vi "VI Konfig FT-IR.vi"() -> ()   [LabVIEW 2020, in "FT-IR.lvlib"]
uses:
  Seiten/FT-IR/FT-IR.lvlib
  Visualisierungs Elemente/Zahlen-Ausgabefeld.ctl
  Visualisierungs Elemente/Zahlen-Eingabefeld.ctl
  Visualisierungs Elemente/String - Ausgabefeld.ctl
  Visualisierungs Elemente/Button.ctl
  Visualisierungs Elemente/Auswahlfeld.ctl
  Seiten/FT-IR/1Hz-5Hz Geraet.ctl
  Seiten/FT-IR/xyGraph.ctl
  Seiten/FT-IR/ReadLabFile/Aswahl Lab File.ctl
  Seiten/FT-IR/FGV FT-IR Diagnose Aktionen.ctl
  Seiten/FT-IR/FGV FT-IR Aktionen.ctl
  Seiten/FT-IR/FGV FT-IR Gasliste Aktionen.ctl
  Passwortverwaltung/FGV Passwort Aktion.ctl
  Seiten/FT-IR/ReadLabFile/Aktionen Lab File.ctl
  Seiten/FT-IR/Aktionen EVID-Codes.ctl
  Seiten/FT-IR/Get Spectra/Aktion FGV Background-Daten.ctl
  Messdaten/Aktionen FGV Messdaten.ctl
  Auto Kalibrieren/Aktionen Zeitstempel speichern.ctl
  Seiten/FT-IR/Span/Aktion FGV Span.ctl
  Seiten/FT-IR/Get Spectra/get Spectra.vi
  Allgemein/Diagnose Zykluszeit.vi
  Seiten/FT-IR/Span/VI Span Seite.vi
  Seiten/FT-IR/Konfig Recipes.vi
  Seiten/FT-IR/Algebraic Modul/VI Algebraic Konfig.vi
  Passwortverwaltung/Passwort.lvlib
  Seiten/FT-IR/TOOLweb Interface Library/TOOLweb Interface.lvlib
  Allgemein/allgemeine Sub-VIs.lvlib
  Seiten/Grafik/Grafik.lvlib
  Messdaten/Messdaten.lvlib
  Seiten/Log Konfig/LogKonfig.lvlib
  Seiten/FT-IR/ReadLabFile/Read Lab File.lvlib
  Seiten/FT-IR/Algebraic Modul/Algebraic Modul.lvlib
  cRIO/PC/Kommunikation mit cRIO.lvlib
  Seiten/FT-IR/Get Spectra/Get Spectra.lvlib
  Seiten/FT-IR/Span/Spanfaktor.lvlib
  Auto Kalibrieren/Auto Kalibrieren.lvlib
panel:
  in  "Algebraic":T1
  in  "Average IAG Software:":bool caption="IAG Software:"
  in  "Average":u32=1 caption="Rolling - Average:" min=1 max=600
  in  "Average via AK:":bool caption="AK:"
  in  "Smoothing Aktiv?:":bool
  in  "Komm. Leitsystem:":T2=1 caption="Komm. Leitsystem" items=["1Hz"=1, "5Hz"=5, "10Hz"=10]
  in  "Span":bool caption="FTIR-Diag"
  in  "Rezepte wechseln":bool caption="FTIR-Diag"
  in  "Diagnose Zykluszeit":bool caption="FTIR-Diag"
  in  "FTIR-Diag":bool
  out "Mwert":sgl format="%.3f"
  out "PMwert":sgl format="%.3f"
  in  "Gas 1":T3 items=["NO (350,3000) LP 191C", "NO2 (150) LP 191C (1of2)", "NO2 (2000) LP 191C (2of2)", "N2O (300) LP 191C (1of2)", "NH3 (300) LP 191C (1of2)", "NH3 (900,3000) LP 191C (2of2)", "HNCO (400) 191C", "H2O% (30) LP 191C", "Formaldehyde (70,500) LP 191C", "CO2 low% (4) LP 191C (2of2)", "CO2% (20) LP 191C (1of2)", "CO (700) LP 191C (1of3)", "CO% (1) LP 191C (2of3)", "Propylene (1000) LP 191C", "Aromatic HC C7 (500) LP 191C", "Ethylene (1000) LP 191C", "CH4 (250) LP 191C (1of2)", "CH4 (5000) LP 191C (2of2)", "Ethane (1000) LP 191C", "Acetylene (1000) LP 191C", "HNO2 (20) 191C", "MeOH (1000) 191C", "CO% (10) LP 191C (3of3)", "Formic Acid (100) 191C", "SO2 (500) LP 191C", "Acetaldehyde (1000) LP 191C", "COS (100) LP 191C", "1,3 butadiene (100) LP 191C", "Oil as Octane (200) LP 191C", "N2O (1000) LP 191C (2of2)", "Propane (200) LP 191C", "NO2 autorange (2000)", "CO autorange (100000)", "CH4 autorange (5000)", "NH3 autorange (3000)", "NOx autorange (3000)", "HCD (10000)", "NMHCD (10000)", "CO2% autorange (20)", "H2Oppm (300000)", "N2O autorange (1000)", "NMNEHCD (3000)", "Temp. Messzelle", "Druck Messzelle", "sBeam@2500", "Temp. HL zu FT-IR", "Temp. HL Extern SP1", "Austrittstemp. FT-IR", "Temp. Schaltschrank", "Konstant 0", "Konstant 50", "Konstant 100", "AK DUMMY"]
  out "Konzentration 1":T4 format="%.3f"
  out "Graph 1":waveform(dbl)(graph)
  in  "Auswahl":T5
  out "Zeitstempel":timestamp
  out "Graph":T6 caption="Graph 2"
  out "Zykluszeit":T4 caption="Zykluszeit:" format="%.3f"
  in  "Gerätetype:":T2=1 items=["1Hz"=1, "5Hz"=5, "10Hz"=10]
  out "Zeitstempeln":timestamp[](array[timestamp]) format="%<%H:%M:%S\n%x>T"
  in  "Anzahl":i32=1
  in  "Startadresse":i32=11000
  out "Betriebsstunden FT-IR":T4 format="%.1f"
  out "Aktuelles Rezept":T7
  in  "Gasliste vergleichen":T1
  out "Aktuelle Gasliste":T7[](array[typedef])
  out "(1) InstrumentState":T7
  in  "(90) ftirScans":T8 format="%#_5g"
  out "(10) NrOfGasses":T4 format="%#_5g"
  in  "FT-IR MAX":T9 {"Max sBeam" format="%#_5g"; "Max LinCheck" format="%#_5g"; "Max LaserPP" format="%#_5g"}
  in  "FT-IR MIN":T10 {"Min sBeam" format="%#_5g"; "Min LinCheck" format="%#_5g"; "Min LaserPP" format="%#_5g"}
  out "Ist sBeam":T4 format="%.2f"
  out "Ist LinCheck":T4 format="%.4f"
  out "Ist LaserPP":T4 format="%.2f"
  # "Konfiguration FT-IR"
  # "Diagnose FT-IR"
  # "Istwert"
  # "Minimaler Wert"
  # "Maximaler Wert"
  # "Aktuelle Gasliste"
  # "Laser PP:"
  # "Linearizer Check:"
  # "sBeam@2500"
  # "Allgemeine Parameter"
  # "Messwerte"
  # "Hintergrund Spectrum"
  # "sec"
  # "±"
  # "x"
  # "Zykluszeit:"
  # "sec"
  # "Letzte Kalibrierung:"
  # "Algebraic (EVID Code):"
  # "Startadresse:"
  # "Anzahl:"
  # "Betriebsstunden FT-IR:"
  # "Aktuelles Rezept:"
  # "Instrument State:"
  # "Number of Scan:"
  # "Number of Gases:"
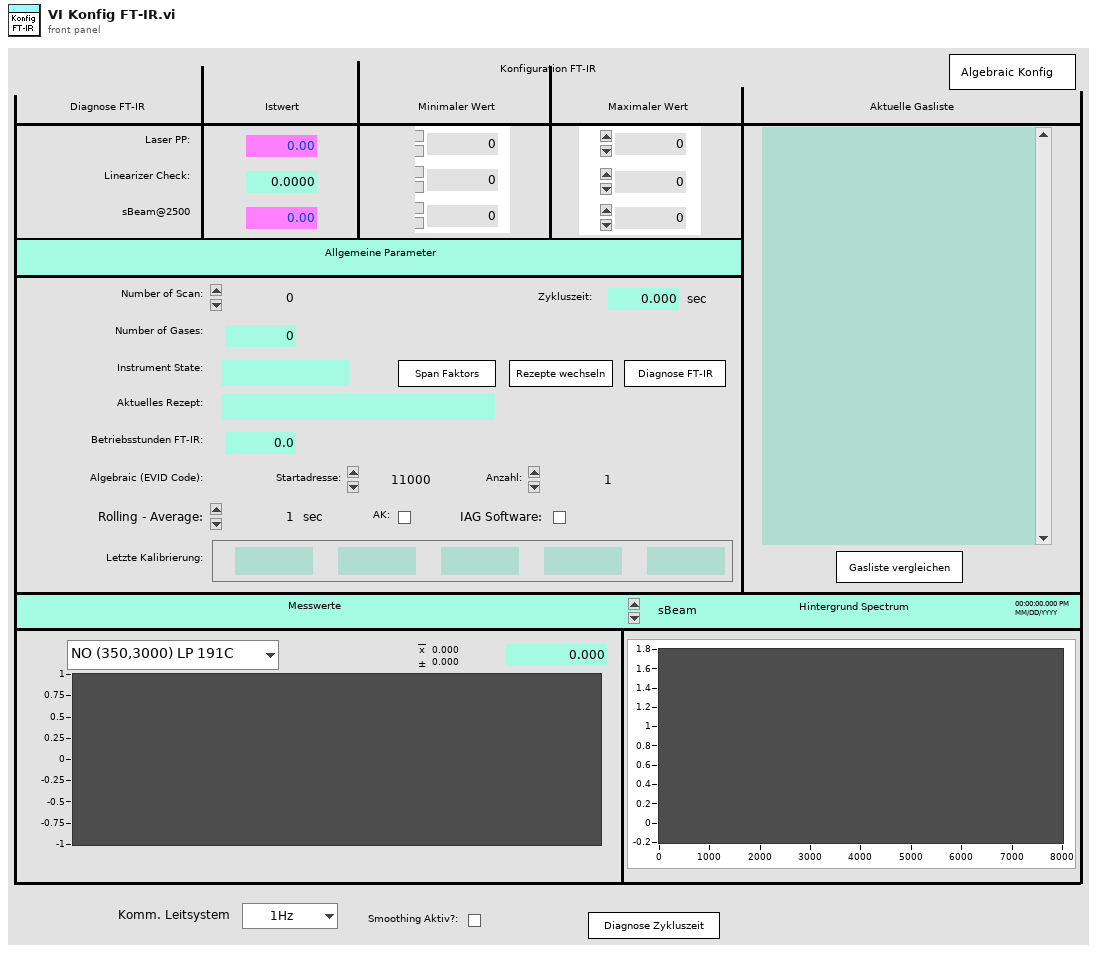
[diagram p1: front panel]
types:
  T1 = typedef "Button.ctl" = bool
  T2 = typedef "FT-IR.lvlib/1Hz-5Hz Geraet.ctl" = u16
  T3 = typedef "Auswahlfeld.ctl" = u16
  T4 = typedef "Zahlen-Ausgabefeld.ctl" = sgl
  T5 = typedef "FT-IR.lvlib/Read Lab File.lvlib/Aswahl Lab File.ctl" = enum16{"sBeam", "Main", "igram", "Previous"}
  T6 = typedef "FT-IR.lvlib/xyGraph.ctl" = cluster{dbl[], "Y":dbl[]}[]
  T7 = typedef "String - Ausgabefeld.ctl" = string
  T8 = typedef "Zahlen-Eingabefeld.ctl" = sgl
  T9 = cluster{"Max LaserPP":T8, "Max LinCheck":T8, "Max sBeam":T8}
  T10 = cluster{"Min LaserPP":T8, "Min LinCheck":T8, "Min sBeam":T8}
  T11 = typedef "FT-IR.lvlib/Get Spectra.lvlib/Aktion FGV Background-Daten.ctl" = enum16{"lesen", "schreiben", "Background aktiv", "Referenz", "laden", "speichern", "Plot sichtbar"}
  T12 = enum8{"Enabled", "Disabled", "Disabled and Grayed Out"}
  T13 = typedef "FT-IR.lvlib/Aktionen EVID-Codes.ctl" = enum16{"lesen", "setzen", "laden", "speichern", "1Hz/5Hz", "Smoothing", "Rolling Average"}
  T14 = typedef "FT-IR.lvlib/Read Lab File.lvlib/Aktionen Lab File.ctl" = enum16{"lesen", "laden"}
  T15 = typedef "Passwort.lvlib/FGV Passwort Aktion.ctl" = enum16{"prüfen", "setzen", "Initialisieren", "PW speichern", "lesen", "PW Änderung"}
  T16 = typedef "FT-IR.lvlib/FGV FT-IR Gasliste Aktionen.ctl" = enum16{"lesen", "Gasliste FT-IR", "Gasliste ausgelesen", "laden", "speichern", "löschen"}
  T17 = typedef "FT-IR.lvlib/FGV FT-IR Aktionen.ctl" = enum16{"lesen", "NOG setzen", "NOS setzen", "Initialisieren", "speichern", "ALLES setzen", "FT-IR Spektrum loggen", "Komm Stoppen", "Spektrum LogKonfig"}
  T18 = typedef "FT-IR.lvlib/FGV FT-IR Diagnose Aktionen.ctl" = enum16{"Lesen", "Diagnose Schreiben", "Min Schreiben", "Max Schreiben"}
  T19 = typedef "FT-IR.lvlib/Rolling Average Settings.ctl" = cluster{"Average":u32, "Average via AK:":bool, "Average IAG Software:":bool}
  T20 = cluster{"LaserPP Max":dbl, "LinCheck Max":dbl, "sBeam Max":dbl}
  T21 = cluster{"LaserPP Min":dbl, "LinCheck Min":dbl, "sBeam Min":dbl}
  T22 = typedef "Auto Kalibrieren.lvlib/Aktionen Zeitstempel speichern.ctl" = enum16{"lesen", "Zeitstempel NEU", "laden", "speichern"}
  T23 = typedef "Messdaten.lvlib/Aktionen FGV Messdaten.ctl" = enum16{"lesen", "schreiben", "löschen", "Mittelwerte", "Komponente"}
  T24 = typedef "FT-IR.lvlib/Spanfaktor.lvlib/Aktion FGV Span.ctl" = enum16{"lesen", "Span", "Seite aktiv", "Offset", "FGV aktualisiert", "Aktualisierung aufheben"}
  T25 = typedef "FT-IR.lvlib/TOOLweb Interface.lvlib/Typdefinitionen.lvlib/TOOLweb Diagnose.ctl" = cluster{"(14) temperature":sgl, "(15) pressure":sgl, "(16) oxygen":sgl, "(50) diag-igramdc":sgl, "(51) diag-igrampp":sgl, "(52) diag-phaseAngle":sgl, "(53) diag-laserpp":sgl, "(54) diag-laserdc":sgl, "(55) diag-badscan":sgl, "(56) diag-centerburst":sgl, "(57) diag-linearizerCheck":sgl, "(58) diag-SNR":sgl, "(59) diag-sBeamIntensity":sgl}
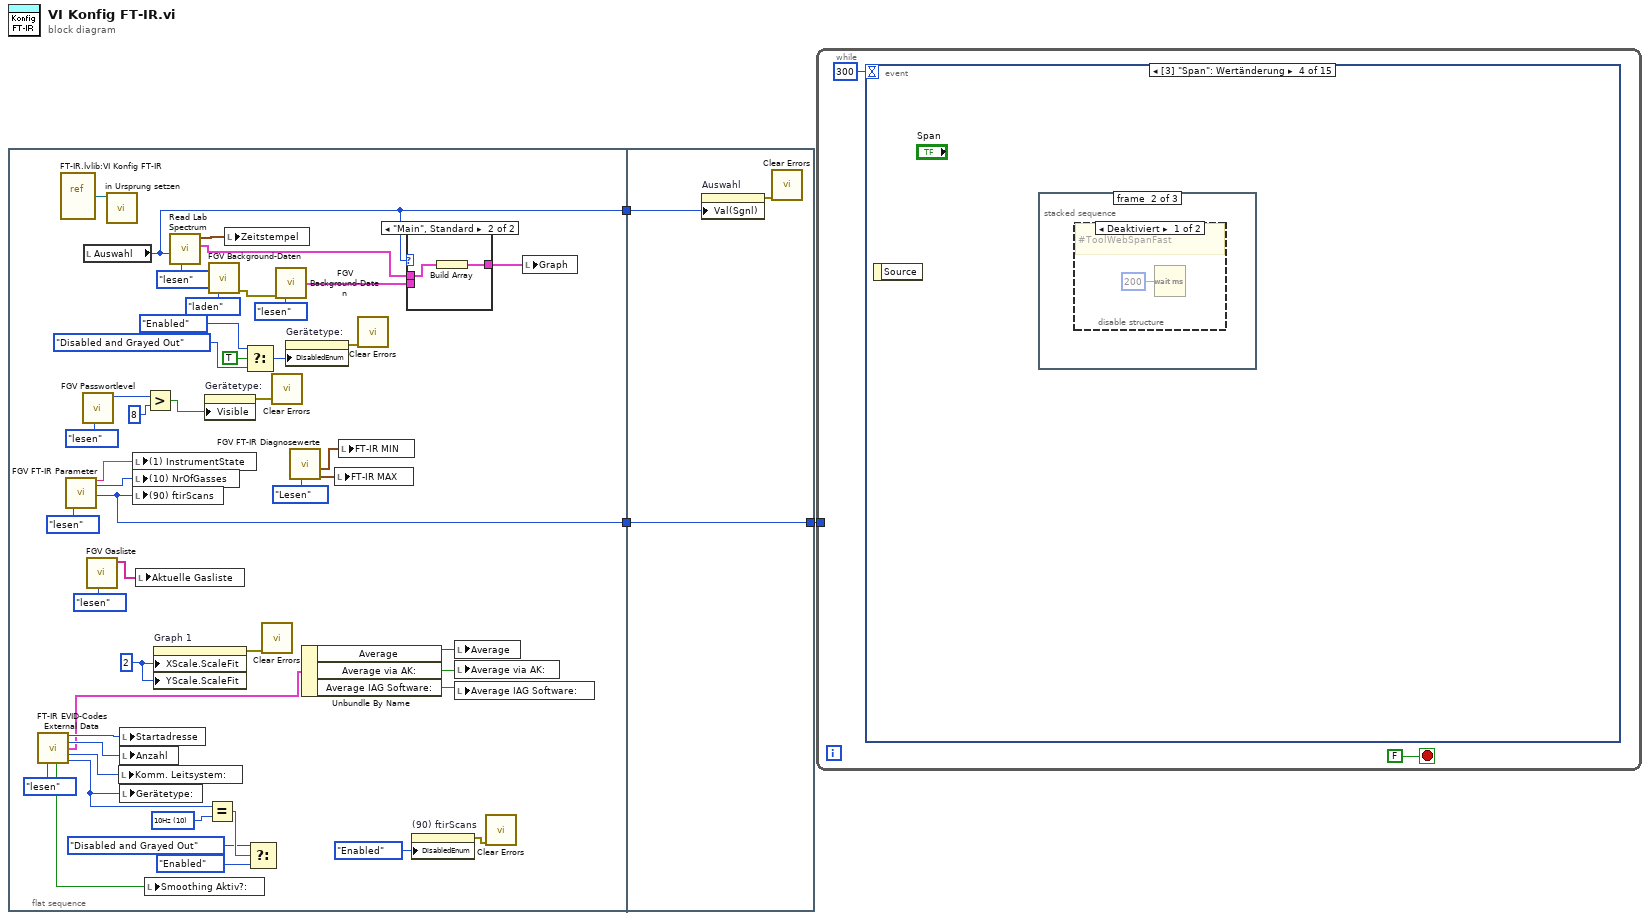
[diagram p0: block diagram]
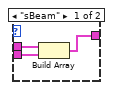
[diagram p2: hidden frame]
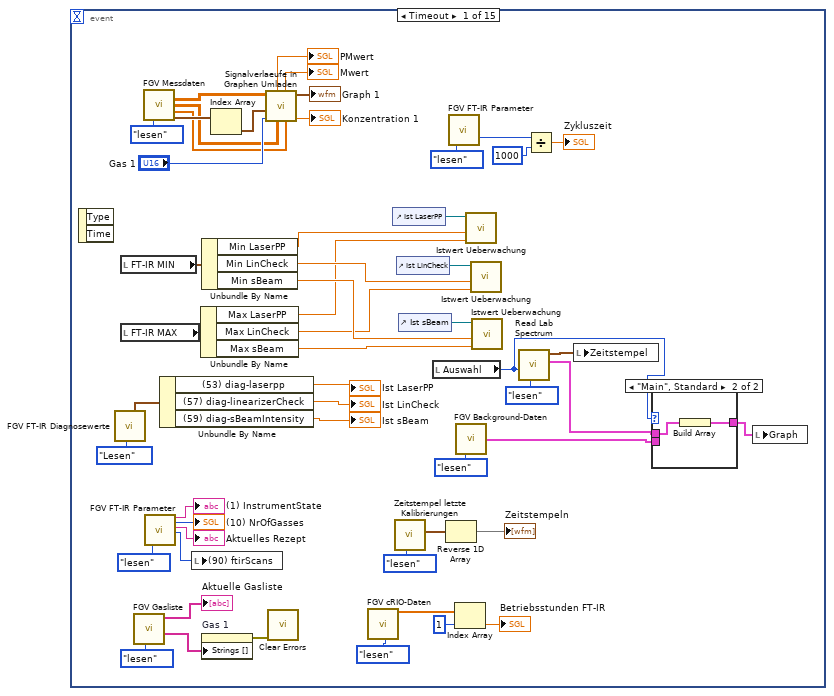
[diagram p3: hidden frame]
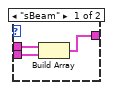
[diagram p4: hidden frame]
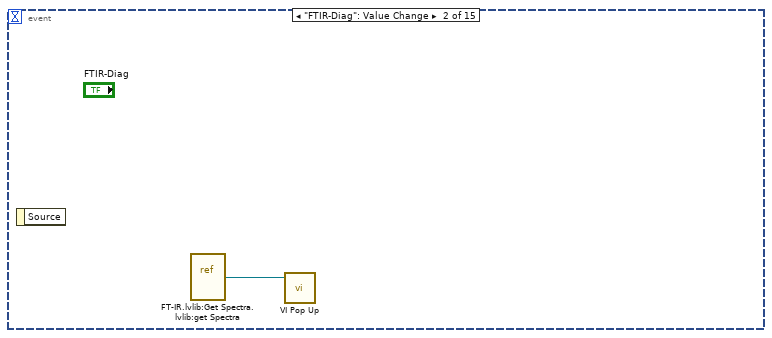
[diagram p5: hidden frame]
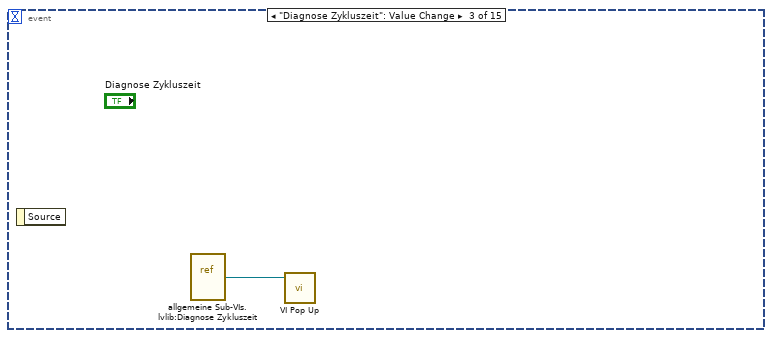
[diagram p6: hidden frame]
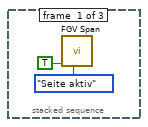
[diagram p7: hidden frame]
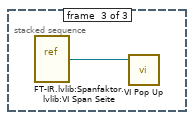
[diagram p9: hidden frame]
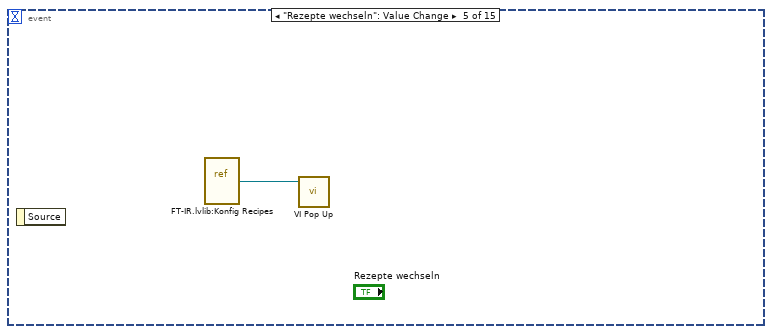
[diagram p10: hidden frame]
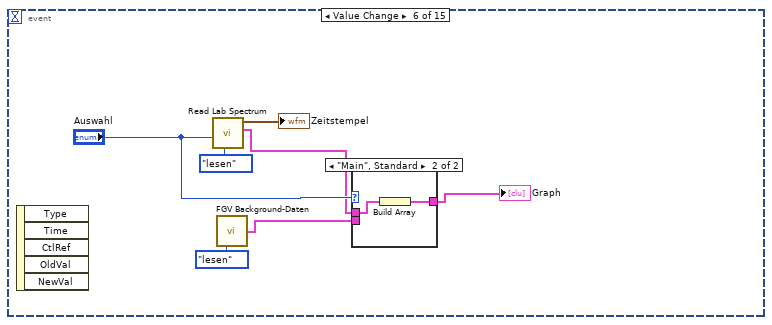
[diagram p11: hidden frame]
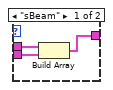
[diagram p12: hidden frame]
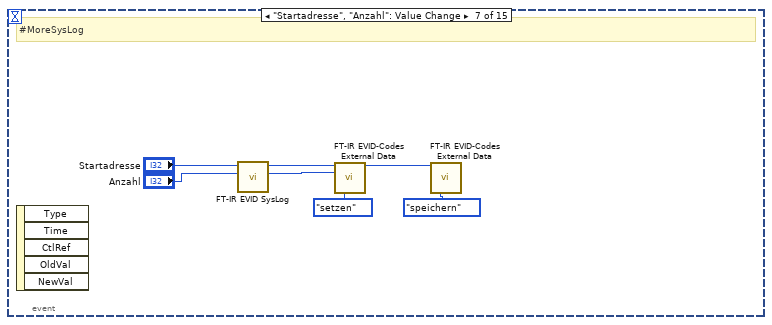
[diagram p13: hidden frame]
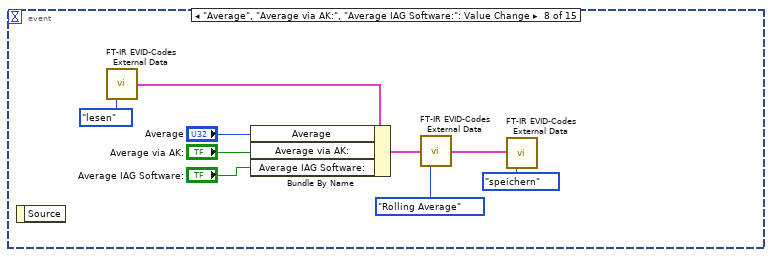
[diagram p14: hidden frame]
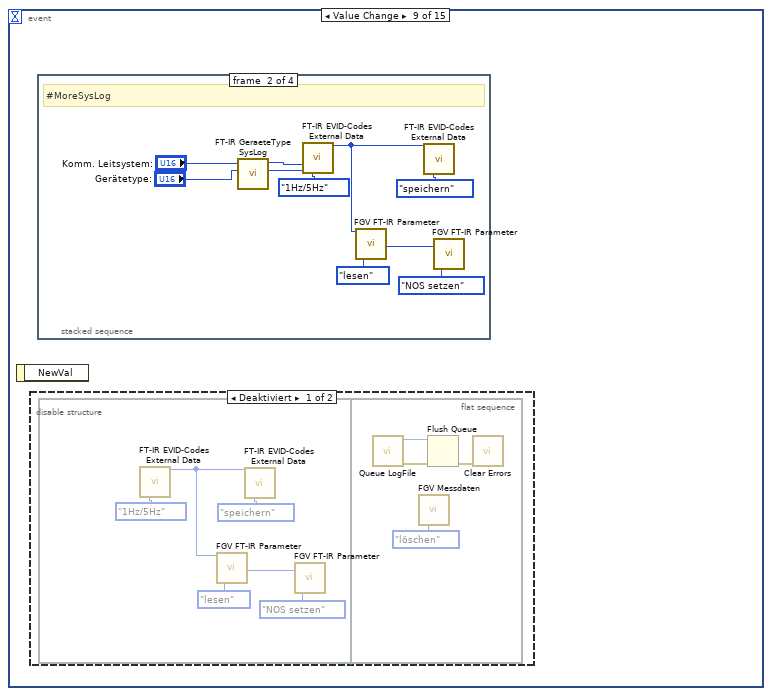
[diagram p15: hidden frame]
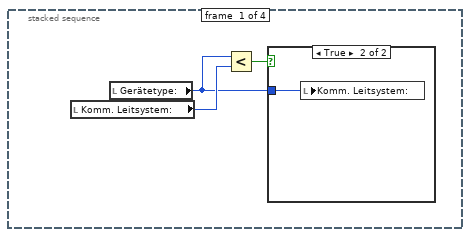
[diagram p17: hidden frame]
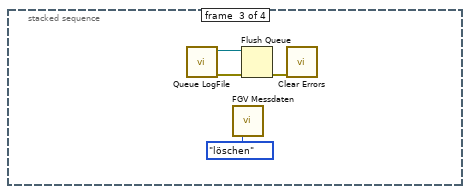
[diagram p19: hidden frame]
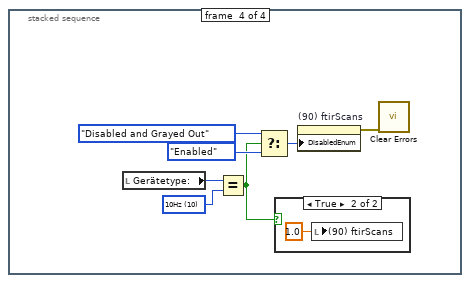
[diagram p20: hidden frame]
diagram:
  n1 = flat-sequence {
    tunnel: [w44] -> w3
    tunnel: [w5] -> w2
    tunnel: [w58] -> w1
    tunnel: w3 -> [w58]
    tunnel: w2 -> [w57]
    frame #0 {
      w23 = T2 10 items=["1Hz"=1, "5Hz"=5, "10Hz"=10] ("y")
      w42 = u8 2 ("X-Achse.Achsenanpassung")
      n2 = call "FT-IR EVID-Codes External Data.vi"("Aktionen"=Aktionen_EVID-Codes."lesen") -> ("Startadresse"=w26:i32, "Anzahl"=w27:i32, "Rolling Average Settings"=w16:T19, "1Hz/5Hz Leitsystem"=w19:T2, "Smoothing?"=w17:bool, "1Hz/5Hz Gerät"=w20:T2)  [unwired: 9 in]
      n3 = vi-ref "FT-IR.lvlib:VI Konfig FT-IR.vi"() -> (w32:refnum<vi>)
      n4 = call "FGV FT-IR Parameter.vi"("Aktion"=FGV_FT-IR_Aktionen."lesen") -> ("Instrument State"=w45:string, "NoOfGasses"=w46:u32, "NoOfScan"=w44:u32)  [unwired: 11 in, 5 out]
      n5 = call "FGV Passwortlevel.vi"("FGV Passwort Aktion"=FGV_Passwort_Aktion."lesen") -> ("aktueller Level"=w40:i16)  [unwired: 3 in, 7 out]
      n6 = local read "Auswahl"() -> (w5:T5)
      n7 = call "FGV Gasliste.vi"("Aktionen"=FGV_FT-IR_Gasliste_Aktionen."lesen") -> ("Aktuelle Gasliste FT-IR"=w30:T7[])  [unwired: 8 in, 2 out]
      n8 = call "in Ursprung setzen.vi"("VI Referenz"=w32) -> ()  [unwired: 10 in, 1 out]
      n9 = local write "Komm. Leitsystem:"(w19) -> ()
      n10 = local write "Startadresse"(w26) -> ()
      n11 = local write "Anzahl"(w27) -> ()
      n12 = local write "Gerätetype:"(w20) -> ()
      n13 = local write "(1) InstrumentState"(w45) -> ()
      n14 = local write "(10) NrOfGasses"(w46) -> ()
      n15 = local write "(90) ftirScans"(w44) -> ()
      n16 = local write "Aktuelle Gasliste"(w30) -> ()
      n17 = Greater?(x=w40, y=i16 8) -> (0:w29:bool)
      n18 = local write "Smoothing Aktiv?:"(w17) -> ()
      n19 = property on="Graph 1" class="SVDiagr (strikt)"("XScale.ScaleFit"=w42, "YScale.ScaleFit"=w42) -> (error out=w36:errorcluster)  [unwired: 2 in, 1 out]
      n20 = call "Read Lab Spectrum.VI"("Aktionen"=Aktionen_Lab_File."lesen", "Auswahl"=w5) -> ("Graph"=w9:cluster{dbl[], sgl[]}, "Zeitstempel"=w12:timestamp)  [unwired: 6 in, 2 out]
      n21 = property on="Gerätetype:" class="Ring (strikt)"("Visible"=w29) -> (error out=w28:errorcluster)  [unwired: 2 in, 1 out]
      n22 = Equal?(x=w20, y=w23) -> (x = y?=w24:bool)
      n23 = call "FGV Background-Daten.vi"("Aktion"=Aktion_FGV_Background-Daten."laden") -> ("error out"=w6:errorcluster)  [unwired: 7 in, 7 out]
      n24 = local write "Zeitstempel"(w12) -> ()
      n25 = Select(t=T12."Enabled", s=TRUE, f=T12."Disabled and Grayed Out" ("Deaktiviert")) -> (s? t:f=w33:T12)
      n26 = Select(t=T12."Disabled and Grayed Out" ("Deaktiviert"), s=w24, f=T12."Enabled" ("t")) -> ()  [unwired: 1 out]
      n27 = call <vilib>:"Clear Errors.vi"("error in (no error)"=w36) -> ()  [unwired: 5 in, 2 out]
      n28 = call <vilib>:"Clear Errors.vi"("error in (no error)"=w28) -> ()  [unwired: 5 in, 2 out]
      n29 = call "FGV Background-Daten.vi"("error in (no error)"=w6, "Aktion"=Aktion_FGV_Background-Daten."lesen") -> ("Referenz-200"=w4:cluster{"Ramp Pattern":dbl[], dbl[]})  [unwired: 6 in, 7 out]
      n30 = property on="Gerätetype:" class="Ring (strikt)"("DisabledEnum"=w33) -> (error out=w37:errorcluster)  [unwired: 2 in, 1 out]
      n31 = call "FGV FT-IR Diagnosewerte.vi"("Aktionen"=FGV_FT-IR_Diagnose_Aktionen."Lesen") -> ("FT-IR MAX"=w50:T20, "FT-IR MIN"=w49:T21)  [unwired: 5 in, 4 out]
      n32 = Unbundle By Name(w16) -> ("Average"=w15:u32, "Average via AK:"=w14:bool, "Average IAG Software:"=w13:bool)
      n33 = local write "FT-IR MAX"(w50) -> ()
      n34 = local write "FT-IR MIN"(w49) -> ()
      n35 = call <vilib>:"Clear Errors.vi"("error in (no error)"=w37) -> ()  [unwired: 5 in, 2 out]
      n36 = case shown="\"Main\", Standard" w5 {
        tunnel: w4 -> [w53 _]
        tunnel: w9 -> [w52 w55]
        tunnel: [w51 w54] -> w8
        frame "sBeam" {
          n37 = Build Array(w52, w53) -> (w51:cluster{"Ramp Pattern":dbl[], dbl[]}[])
        }
        frame "Main", Default {
          n38 = Build Array(w55) -> (w54:cluster{dbl[], sgl[]}[])
        }
      }
      n39 = property on="(90) ftirScans" class="DigWert (strikt)"("DisabledEnum"=T12."Enabled" ("Deaktiviert")) -> (error out=w18:errorcluster)  [unwired: 2 in, 1 out]
      n40 = local write "Average"(w15) -> ()
      n41 = local write "Average via AK:"(w14) -> ()
      n42 = local write "Average IAG Software:"(w13) -> ()
      n43 = call <vilib>:"Clear Errors.vi"("error in (no error)"=w18) -> ()  [unwired: 5 in, 2 out]
      n44 = local write "Graph"(w8) -> ()
    }
    frame #1 {
      n45 = property on="Auswahl" class="Enum (strikt)"("Val(Sgnl)"=w57) -> (error out=w56:errorcluster)  [unwired: 2 in, 1 out]
      n46 = call <vilib>:"Clear Errors.vi"("error in (no error)"=w56) -> ()  [unwired: 5 in, 2 out]
    }
  }
  n47 = while {
    tunnel: w1 -> [_]
    stop <- FALSE stop-if-true
    n48 = event shown="[3] \"Span\": Wertänderung" {
      selector: _ -> [_ _ _ _ _ _ _ _ _ _ _ _ _ _ _]
      dyn-events: _ -> [_ _ _ _ _ _ _ _ _ _ _ _ _ _ _]
      timeout: 300 -> [_ _ _ _ _ _ _ _ _ _ _ _ _ _ _]
      event Timeout {
        n49 = event-data() -> ()  [unwired: 1 in, 2 out]
        n50 = call "FGV FT-IR Diagnosewerte.vi"("Aktionen"=FGV_FT-IR_Diagnose_Aktionen."Lesen") -> ("Diagnose"=w103:T25)  [unwired: 5 in, 5 out]
        n51 = local read "FT-IR MIN"() -> (w107:T10)
        n52 = local read "FT-IR MAX"() -> (w108:T9)
        n53 = call "FGV Gasliste.vi"("Aktionen"=FGV_FT-IR_Gasliste_Aktionen."lesen") -> ("Aktuelle Gasliste gesamt"=w73:T7[], "Aktuelle Gasliste FT-IR"=→"Aktuelle Gasliste":T7[])  [unwired: 8 in, 1 out]
        n54 = call "FGV Messdaten.vi"("Aktionen"=Aktionen_FGV_Messdaten."lesen") -> ("Messdaten"=w74:sgl[][], "Mittelwertdaten"=w72:sgl[][], "Deviation"=w71:sgl[], "Zeitstempeln"=w88:timestamp[])  [unwired: 6 in, 5 out]
        n55 = call "FGV FT-IR Parameter.vi"("Aktion"=FGV_FT-IR_Aktionen."lesen") -> ("Instrument State"=→"(1) InstrumentState":string, "NoOfGasses"=→"(10) NrOfGasses":u32, "Current Recipe"=→"Aktuelles Rezept":string, "NoOfScan"=w68:u32)  [unwired: 11 in, 4 out]
        n56 = Unbundle By Name(w103) -> ("(53) diag-laserpp"=→"Ist LaserPP":sgl, "(57) diag-linearizerCheck"=→"Ist LinCheck":sgl, "(59) diag-sBeamIntensity"=→"Ist sBeam":sgl)
        n57 = local write "(90) ftirScans"(w68) -> ()
        n58 = Unbundle By Name(w108) -> ("Max LaserPP"=w110:T8, "Max LinCheck"=w112:T8, "Max sBeam"=w114:T8)
        n59 = Unbundle By Name(w107) -> ("Min LaserPP"=w109:T8, "Min LinCheck"=w111:T8, "Min sBeam"=w113:T8)
        n60 = property on="Gas 1" class="Ring (strikt)"("Strings []"=w73) -> (error out=w75:errorcluster)  [unwired: 2 in, 1 out]
        n61 = Index Array(array=w88) -> (element=w86:timestamp)  [unwired: 1 in]
        n62 = call "Signalverlaeufe in Graphen Umladen.vi"("Deviation"=w71, "Mittelwertdaten"=w72, "Gas-Auswahl"="Gas 1", "t0"=w86, "Werte"=w74) -> ("Konzentration"=→"Konzentration 1":sgl, "Waveform"=→"Graph 1":waveform(dbl), "aktuelle Mittelwert"=→"Mwert":sgl, "Deviation"=→"PMwert":sgl)  [unwired: 2 in, 1 out]
        n63 = call <vilib>:"Clear Errors.vi"("error in (no error)"=w75) -> ()  [unwired: 5 in, 2 out]
        n64 = call "FGV cRIO-Daten.vi"("Aktion"=enum16{"lesen", "schreiben"}."lesen") -> ("Betriebsstunden"=w76:sgl[])  [unwired: 9 in, 9 out]
        n65 = control-ref of="Ist LaserPP"() -> (w104:refnum<vi>)
        n66 = call "Zeitstempel letzte Kalibrierungen.vi"("Aktionen"=Aktionen_Zeitstempel_speichern."lesen") -> ("Zeitstempeln"=w66:timestamp[])  [unwired: 10 in]
        n67 = control-ref of="Ist LinCheck"() -> (w105:refnum<vi>)
        n68 = control-ref of="Ist sBeam"() -> (w106:refnum<vi>)
        n69 = local read "Auswahl"() -> (w62:T5)
        n70 = Reverse 1D Array(array=w66) -> (reversed array=→"Zeitstempeln":timestamp[])
        n71 = call "FGV FT-IR Parameter.vi"("Aktion"=FGV_FT-IR_Aktionen."lesen") -> ("Zykluszeit Messdatenverteiler"=w82:u32)  [unwired: 11 in, 7 out]
        n72 = Index Array(array=w76, index=1 ("Index")) -> (element=→"Betriebsstunden FT-IR":sgl)
        n73 = call "FGV Background-Daten.vi"("Aktion"=Aktion_FGV_Background-Daten."lesen") -> ("Referenz-200"=w61:cluster{"Ramp Pattern":dbl[], dbl[]})  [unwired: 7 in, 7 out]
        n74 = call "Istwert Ueberwachung.vi"("Max"=w110, "Min"=w109, "Referernz"=w104) -> ()  [unwired: 9 in]
        n75 = call "Istwert Ueberwachung.vi"("Max"=w112, "Min"=w111, "Referernz"=w105) -> ()  [unwired: 9 in]
        n76 = call "Istwert Ueberwachung.vi"("Max"=w114, "Min"=w113, "Referernz"=w106) -> ()  [unwired: 9 in]
        n77 = call "Read Lab Spectrum.VI"("Aktionen"=Aktionen_Lab_File."lesen", "Auswahl"=w62) -> ("Graph"=w64:cluster{dbl[], sgl[]}, "Zeitstempel"=w70:timestamp)  [unwired: 6 in, 2 out]
        n78 = Divide(x=w82, y=u32 1000) -> (x/y=→"Zykluszeit":dbl)
        n79 = local write "Zeitstempel"(w70) -> ()
        n80 = case shown="\"Main\", Standard" w62 {
          tunnel: w61 -> [w117 _]
          tunnel: w64 -> [w116 w119]
          tunnel: [w115 w118] -> w63
          frame "sBeam" {
            n81 = Build Array(w116, w117) -> (w115:cluster{"Ramp Pattern":dbl[], dbl[]}[])
          }
          frame "Main", Default {
            n82 = Build Array(w119) -> (w118:cluster{dbl[], sgl[]}[])
          }
        }
        n83 = local write "Graph"(w63) -> ()
      }
      event "FTIR-Diag": Value Change {
        n84 = event-data() -> ()  [unwired: 1 in, 1 out]
        n85 = vi-ref "FT-IR.lvlib:Get Spectra.lvlib:get Spectra.vi"() -> (w120:refnum<vi>)
        n86 = call "VI Pop Up.vi"("VI Referenz"=w120) -> ()  [unwired: 10 in, 1 out]
      }
      event "Diagnose Zykluszeit": Value Change {
        n87 = event-data() -> ()  [unwired: 1 in, 1 out]
        n88 = vi-ref "allgemeine Sub-VIs.lvlib:Diagnose Zykluszeit.vi"() -> (w121:refnum<vi>)
        n89 = call "VI Pop Up.vi"("VI Referenz"=w121) -> ()  [unwired: 10 in, 1 out]
      }
      event "Span": Value Change {
        n90 = event-data() -> ()  [unwired: 1 in, 1 out]
        n91 = stacked-sequence {
          frame #0 {
            n92 = call "FGV Span.vi"("Aktion"=Aktion_FGV_Span."Seite aktiv", "Aktiv"=TRUE) -> ()  [unwired: 6 in, 4 out]
          }
          frame #1 {
            n93 = disable-structure shown="Deaktiviert" {
              frame Disabled {
                # "#ToolWebSpanFast"
                n94 = Wait (ms)(milliseconds to wait=u32 200 ("Zu wartende ms")) -> ()  [unwired: 1 out]
              }
              frame Enabled {
              }
            }
          }
          frame #2 {
            n95 = vi-ref "FT-IR.lvlib:Spanfaktor.lvlib:VI Span Seite.vi"() -> (w125:refnum<vi>)
            n96 = call "VI Pop Up.vi"("VI Referenz"=w125) -> ()  [unwired: 10 in, 1 out]
          }
        }
      }
      event "Rezepte wechseln": Value Change {
        n97 = event-data() -> ()  [unwired: 1 in, 1 out]
        n98 = vi-ref "FT-IR.lvlib:Konfig Recipes.vi"() -> (w126:refnum<vi>)
        n99 = call "VI Pop Up.vi"("VI Referenz"=w126) -> ()  [unwired: 10 in, 1 out]
      }
      event Value Change {
        n100 = event-data() -> ()  [unwired: 1 in, 5 out]
        n101 = call "Read Lab Spectrum.VI"("Aktionen"=Aktionen_Lab_File."lesen", "Auswahl"="Auswahl") -> ("Graph"=w130:cluster{dbl[], sgl[]}, "Zeitstempel"=→"Zeitstempel":timestamp)  [unwired: 6 in, 2 out]
        n102 = call "FGV Background-Daten.vi"("Aktion"=Aktion_FGV_Background-Daten."lesen") -> ("Referenz-200"=w127:cluster{"Ramp Pattern":dbl[], dbl[]})  [unwired: 7 in, 7 out]
        n103 = case shown="\"Main\", Standard" "Auswahl" {
          tunnel: w127 -> [w136 _]
          tunnel: w130 -> [w135 w138]
          tunnel: [w134 w137] -> w128
          frame "sBeam" {
            n104 = Build Array(w135, w136) -> (w134:cluster{"Ramp Pattern":dbl[], dbl[]}[])
          }
          frame "Main", Default {
            n105 = Build Array(w138) -> (w137:cluster{dbl[], sgl[]}[])
          }
        }
        "Graph" <- w128
      }
      event "Startadresse", "Anzahl": Value Change {
        # "#MoreSysLog"
        n106 = event-data() -> ()  [unwired: 1 in, 5 out]
        n107 = call "FT-IR EVID SysLog.vi"("Anzahl"="Anzahl", "Startadresse"="Startadresse") -> ("Anzahl out"=w139:i32, "Startadresse out"=w141:i32)  [unwired: 8 in]
        n108 = call "FT-IR EVID-Codes External Data.vi"("Startadresse"=w141, "Anzahl"=w139, "Aktionen"=Aktionen_EVID-Codes."setzen") -> ("Startadresse"=w143:i32)  [unwired: 7 in, 5 out]
        n109 = call "FT-IR EVID-Codes External Data.vi"("Startadresse"=w143, "Aktionen"=Aktionen_EVID-Codes."speichern") -> ()  [unwired: 8 in, 6 out]
      }
      event "Average", "Average via AK:", "Average IAG Software:": Value Change {
        n110 = event-data() -> ()  [unwired: 1 in, 1 out]
        n111 = call "FT-IR EVID-Codes External Data.vi"("Aktionen"=Aktionen_EVID-Codes."lesen") -> ("Rolling Average Settings"=w153:T19)  [unwired: 9 in, 5 out]
        n112 = Bundle By Name(cluster=w153, "Average"="Average", "Average via AK:"="Average via AK:", "Average IAG Software:"="Average IAG Software:") -> (w148:T19)
        n113 = call "FT-IR EVID-Codes External Data.vi"("Rolling Average Settings"=w148, "Aktionen"=Aktionen_EVID-Codes."Rolling Average") -> ("Rolling Average Settings"=w146:T19)  [unwired: 8 in, 5 out]
        n114 = call "FT-IR EVID-Codes External Data.vi"("Rolling Average Settings"=w146, "Aktionen"=Aktionen_EVID-Codes."speichern") -> ()  [unwired: 8 in, 6 out]
      }
      event Value Change {
        n115 = event-data() -> ()  [unwired: 1 in, 1 out]
        n116 = disable-structure shown="Deaktiviert" {
          frame Disabled {
            n117 = flat-sequence {
              frame #0 {
                n118 = call "FT-IR EVID-Codes External Data.vi"("Aktionen"=Aktionen_EVID-Codes."1Hz/5Hz") -> ("Startadresse"=w155:i32)  [unwired: 9 in, 5 out]
                n119 = call "FGV FT-IR Parameter.vi"("NoOfGasses neu"=w155, "Aktion"=FGV_FT-IR_Aktionen."lesen") -> ("NoOfScan"=w156:u32)  [unwired: 10 in, 7 out]
                n120 = call "FT-IR EVID-Codes External Data.vi"("Startadresse"=w155, "Aktionen"=Aktionen_EVID-Codes."speichern") -> ()  [unwired: 8 in, 6 out]
                n121 = call "FGV FT-IR Parameter.vi"("NoOfScan neu"=w156, "Aktion"=FGV_FT-IR_Aktionen."NOS setzen") -> ()  [unwired: 10 in, 8 out]
              }
              frame #1 {
                n122 = call "Queue LogFile.vi"() -> ("error out"=w162:errorcluster, "Queue (Ausgang)"=w163:refnum<queue>)  [unwired: 6 in]
                n123 = call "FGV Messdaten.vi"("Aktionen"=Aktionen_FGV_Messdaten."löschen") -> ()  [unwired: 6 in, 9 out]
                n124 = Flush Queue(queue=w163, error in (no error)=w162) -> (error out=w161:errorcluster)  [unwired: 2 out]
                n125 = call <vilib>:"Clear Errors.vi"("error in (no error)"=w161) -> ()  [unwired: 5 in, 2 out]
              }
            }
          }
          frame Enabled {
          }
        }
        n126 = stacked-sequence {
          frame #0 {
            n127 = local read "Komm. Leitsystem:"() -> (w167:T2)
            n128 = local read "Gerätetype:"() -> (w165:T2)
            n129 = Less?(x=w165, y=w167) -> (x < y?=w166:bool)
            n130 = case shown="True" w166 {
              tunnel: w165 -> [_ w168]
              frame False {
              }
              frame True {
                n131 = local write "Komm. Leitsystem:"(w168) -> ()
              }
            }
          }
          frame #1 {
            # "#MoreSysLog"
            n132 = call "FT-IR GeraeteType SysLog.vi"("Gerätetype:"="Gerätetype:", "Komm. Leitsystem:"="Komm. Leitsystem:") -> ("Gerätetype: out"=w169:T2, "Komm. Leitsystem: out"=w171:T2)  [unwired: 4 in, 2 out]
            n133 = call "FT-IR EVID-Codes External Data.vi"("1Hz/5Hz Leitsystem"=w171, "1Hz/5Hz Gerät"=w169, "Aktionen"=Aktionen_EVID-Codes."1Hz/5Hz") -> ("Startadresse"=w173:i32)  [unwired: 7 in, 5 out]
            n134 = call "FGV FT-IR Parameter.vi"("NoOfGasses neu"=w173, "Aktion"=FGV_FT-IR_Aktionen."lesen") -> ("NoOfScan"=w174:u32)  [unwired: 10 in, 7 out]
            n135 = call "FT-IR EVID-Codes External Data.vi"("Startadresse"=w173, "Aktionen"=Aktionen_EVID-Codes."speichern") -> ()  [unwired: 8 in, 6 out]
            n136 = call "FGV FT-IR Parameter.vi"("NoOfScan neu"=w174, "Aktion"=FGV_FT-IR_Aktionen."NOS setzen") -> ()  [unwired: 10 in, 8 out]
          }
          frame #2 {
            n137 = call "Queue LogFile.vi"() -> ("error out"=w180:errorcluster, "Queue (Ausgang)"=w181:refnum<queue>)  [unwired: 6 in]
            n138 = call "FGV Messdaten.vi"("Aktionen"=Aktionen_FGV_Messdaten."löschen") -> ()  [unwired: 6 in, 9 out]
            n139 = Flush Queue(queue=w181, error in (no error)=w180) -> (error out=w179:errorcluster)  [unwired: 2 out]
            n140 = call <vilib>:"Clear Errors.vi"("error in (no error)"=w179) -> ()  [unwired: 5 in, 2 out]
          }
          frame #3 {
            w188 = T2 10 items=["1Hz"=1, "5Hz"=5, "10Hz"=10] ("y")
            n141 = local read "Gerätetype:"() -> (w189:T2)
            n142 = Equal?(x=w189, y=w188) -> (x = y?=w185:bool)
            n143 = Select(t=T12."Disabled and Grayed Out" ("Deaktiviert"), s=w185, f=T12."Enabled" ("t")) -> (s? t:f=w183:T12)
            n144 = case shown="True" w185 {
              frame False {
              }
              frame True {
                n145 = local write "(90) ftirScans"(T8 1.0 ("(90) ftirScans")) -> ()
              }
            }
            n146 = property on="(90) ftirScans" class="DigWert (strikt)"("DisabledEnum"=w183) -> (error out=w184:errorcluster)  [unwired: 2 in, 1 out]
            n147 = call <vilib>:"Clear Errors.vi"("error in (no error)"=w184) -> ()  [unwired: 5 in, 2 out]
          }
        }
      }
      event "Smoothing Aktiv?:": Value Change {
        n148 = event-data() -> ()  [unwired: 1 in, 6 out]
        n149 = flat-sequence {
          frame #0 {
            n150 = call "FT-IR EVID-Codes External Data.vi"("Smoothing?"="Smoothing Aktiv?:", "Aktionen"=Aktionen_EVID-Codes."Smoothing") -> ("Startadresse"=w192:i32)  [unwired: 8 in, 5 out]
            n151 = call "FT-IR EVID-Codes External Data.vi"("Startadresse"=w192, "Aktionen"=Aktionen_EVID-Codes."speichern") -> ()  [unwired: 8 in, 6 out]
          }
          frame #1 {
            n152 = vi-ref "TOOLweb Rezept wechseln.vi"() -> (w195:refnum<vi>)
            n153 = call "VI Pop Up.vi"("VI Referenz"=w195) -> ()  [unwired: 10 in, 1 out]
          }
        }
      }
      event Value Change {
        n154 = event-data() -> ()  [unwired: 1 in, 1 out]
        n155 = call "FGV Gasliste.vi"("Aktionen"=FGV_FT-IR_Gasliste_Aktionen."lesen") -> ("Gasliste ausgelesen"=w200:T7[], "Aktuelle Gasliste FT-IR"=w201:T7[])  [unwired: 8 in, 1 out]
        n156 = for {
          tunnel: w201 -> [w206] mode=indexing
          tunnel: w200 -> [w205] mode=indexing
          tunnel: [w204] -> w198
          stop <- w204 stop-if-true
          n157 = Not Equal?(x=w206, y=w205) -> (x != y?=w204:bool)
        }
        n158 = Array Size(array=w201) -> (size(s)=w202:i32)
        n159 = Array Size(array=w200) -> (size(s)=w203:i32)
        n160 = Not Equal?(x=w202, y=w203) -> (x != y?=w199:bool)
        n161 = Or(x=w199, y=w198) -> (x .or. y?=w197:bool)
        n162 = call "Gasliste vergleichen.vi"("FT-IR"=w197) -> ()  [unwired: 11 in]
      }
      event "FT-IR MIN": Value Change {
        n163 = event-data() -> ("NewVal"=w208:T10, "OldVal"=w207:T10)  [unwired: 1 in]
        n164 = call "FGV Passwortlevel.vi"("FGV Passwort Aktion"=FGV_Passwort_Aktion."prüfen", "geforderter Level"=i16 8) -> ("Freigabe"=w210:bool)  [unwired: 2 in, 7 out]
        n165 = case shown="True" w210 {
          tunnel: w208 -> [_ w214]
          tunnel: w207 -> [w212 _]
          frame False {
            n166 = local write "FT-IR MIN"(w212) -> ()
          }
          frame True {
            # "#MoreSysLog"
            n167 = call "FT-IR Min SysLog.vi"("NewVal"=w214) -> ("NewVal out"=w213:T10)  [unwired: 10 in]
            n168 = call "FGV FT-IR Diagnosewerte.vi"("Aktionen"=FGV_FT-IR_Diagnose_Aktionen."Min Schreiben", "FT-IR MIN"=w213) -> ()  [unwired: 4 in, 6 out]
          }
        }
      }
      event "FT-IR MAX": Value Change {
        n169 = event-data() -> ("NewVal"=w217:T9, "OldVal"=w216:T9)  [unwired: 1 in]
        n170 = call "FGV Passwortlevel.vi"("FGV Passwort Aktion"=FGV_Passwort_Aktion."prüfen", "geforderter Level"=i16 8) -> ("Freigabe"=w219:bool)  [unwired: 2 in, 7 out]
        n171 = case shown="True" w219 {
          tunnel: w217 -> [_ w223]
          tunnel: w216 -> [w221 _]
          frame False {
            n172 = local write "FT-IR MAX"(w221) -> ()
          }
          frame True {
            # "#MoreSysLog"
            n173 = call "FT-IR Max SysLog.vi"("NewVal"=w223) -> ("NewVal out"=w222:T9)  [unwired: 10 in]
            n174 = call "FGV FT-IR Diagnosewerte.vi"("Aktionen"=FGV_FT-IR_Diagnose_Aktionen."Max Schreiben", "FT-IR MAX"=w222) -> ()  [unwired: 4 in, 6 out]
          }
        }
      }
      event Value Change {
        n175 = event-data() -> ("NewVal"=w226:T8, "OldVal"=w225:T8)  [unwired: 1 in]
        n176 = call "FGV Passwortlevel.vi"("FGV Passwort Aktion"=FGV_Passwort_Aktion."prüfen", "geforderter Level"=i16 8) -> ("Freigabe"=w227:bool)  [unwired: 2 in, 7 out]
        n177 = case shown="True" w227 {
          tunnel: w226 -> [_ _]
          tunnel: w225 -> [w230 _]
          frame False {
            n178 = local write "(90) ftirScans"(w230) -> ()
          }
          frame True {
            n179 = stacked-sequence {
              frame #0 {
                # "#MoreSysLog"
                n180 = call "FT-IR Scans SysLog.vi"("(90) ftirScans"="(90) ftirScans") -> ("(90) ftirScans out"=w231:T8)  [unwired: 10 in]
                n181 = call "FGV FT-IR Parameter.vi"("NoOfScan neu"=w231, "Aktion"=FGV_FT-IR_Aktionen."NOS setzen") -> ("NoOfScan"=w233:u32)  [unwired: 10 in, 7 out]
                n182 = call "TOOLweb SET ftirScans.vi"("ftirScans"=w233) -> ()  [unwired: 2 in, 5 out]
              }
              frame #1 {
                n183 = call "Queue LogFile.vi"() -> ("error out"=w237:errorcluster, "Queue (Ausgang)"=w236:refnum<queue>)  [unwired: 6 in]
                n184 = call "FGV Messdaten.vi"("Aktionen"=Aktionen_FGV_Messdaten."löschen") -> ()  [unwired: 6 in, 9 out]
                n185 = Flush Queue(queue=w236, error in (no error)=w237) -> ()  [unwired: 3 out]
              }
            }
          }
        }
      }
      event Value Change {
        n186 = event-data() -> ()  [unwired: 1 in, 1 out]
        n187 = call "FGV Passwortlevel.vi"("FGV Passwort Aktion"=FGV_Passwort_Aktion."prüfen", "geforderter Level"=i16 8) -> ("Freigabe"=w239:bool)  [unwired: 2 in, 7 out]
        n188 = case shown="True" w239 {
          frame False {
          }
          frame True {
            n189 = vi-ref "FT-IR.lvlib:Algebraic Modul.lvlib:VI Algebraic Konfig.vi"() -> (w241:refnum<vi>)
            n190 = call "VI Pop Up.vi"("VI Referenz"=w241) -> ()  [unwired: 10 in, 1 out]
          }
        }
      }
    }
  }
